vi "addToPaths.vi"(8 "error in (no error)":errorcluster, 10 "Path":path, 11 "ImageStreamViewer in":refnum<class "ImageStreamViewer.lvclass">) -> (0 "error out":errorcluster, 3 "ImageStreamViewer out":refnum<class "ImageStreamViewer.lvclass">)   [LabVIEW 2009, in "Views.lvlib" / "Camera.lvlib" / "ImageStreamViewer.lvclass"]
uses:
  ImageStreamViewer.lvclass
  ImageStreamViewer.lvclass/ImageStreamViewer.ctl
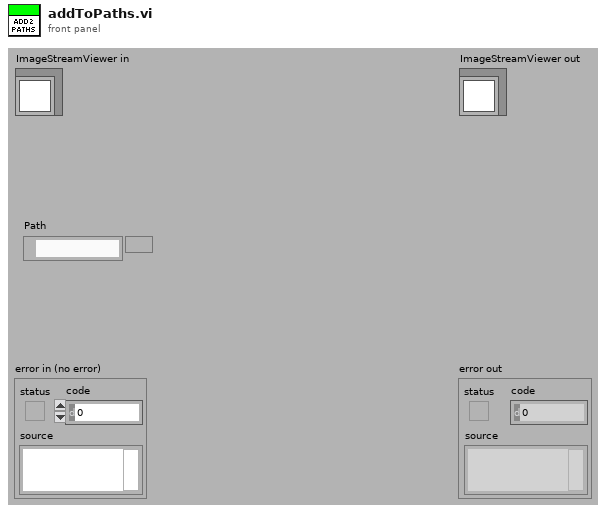
[diagram p1: front panel]
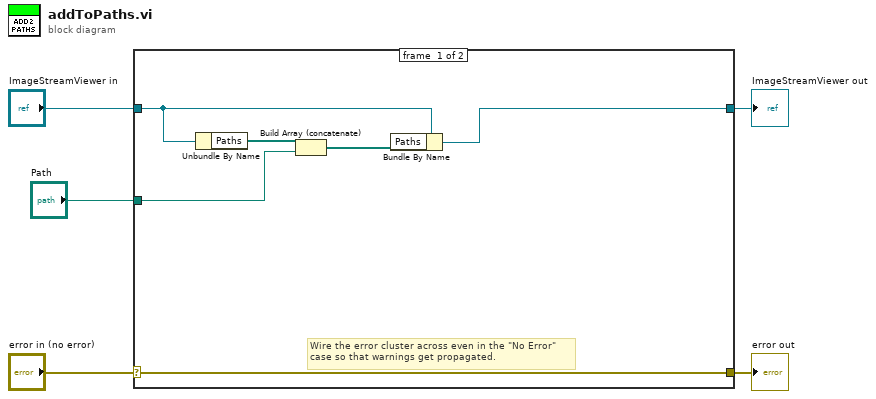
[diagram p0: block diagram]
diagram:
  n1 = case shown="No Error" "error in (no error)" {
    selector: "error in (no error)" -> [w11 w13]
    tunnel: [w11 w13] -> w4
    tunnel: [w6 w12] -> w2
    tunnel: "ImageStreamViewer in" -> [w7 w12]
    tunnel: "Path" -> [w9 _]
    frame #0 {
      # "Wire the error cluster across even in the \"No Error\"\ncase so that warnings get propagated."
      n2 = Unbundle By Name(w7) -> ("Paths"=w10:path[])
      n3 = Build Array (concatenate)(w10, w9) -> (w8:path[])
      n4 = Bundle By Name(cluster=w7, "Paths"=w8) -> (w6:refnum<class "ImageStreamViewer.lvclass">)
    }
    frame #1 {
    }
  }
  "error out" <- w4
  "ImageStreamViewer out" <- w2
